vi "SFOAE-Create Swept Stimuli.vi"(0 "SFOAE Stim":T1, 5 "Data Folder":path, 9 "Fs (Hz)":dbl, 11 "error in (no error)":errorcluster) -> (4 "probe":dbl[](array[numeric]), 6 "suppressor":dbl[](array[numeric]), 8 "offset":i32, 10 "nfft":i32, 15 "error out":errorcluster)   [LabVIEW 2020]
uses:
  Typedefs/SFOAE-Stimulus Parameters.ctl
  Typedefs/SFOAE-Sweep Params.ctl
  epl-vi-lib/Utility VIs/Type Defs/Speaker ring.ctl
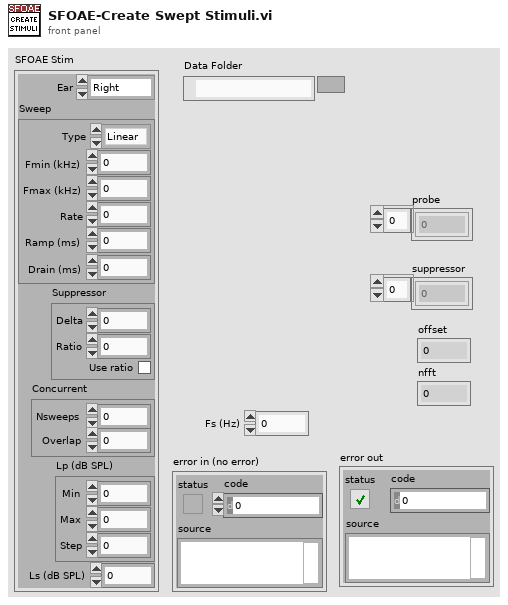
[diagram p1: front panel]
types:
  T1 = typedef "SFOAE-Stimulus Parameters.ctl" = cluster{"Ear":enum16{"Right", "Left"}, "Sweep":T2, "Suppressor":cluster{"Delta":dbl, "Ratio":dbl, "Use ratio":bool}, "Concurrent":cluster{"Nsweeps":i32, "Overlap":dbl}, "Ls (dB SPL)":dbl, "Lp (dB SPL)":cluster{"Min":dbl, "Max":dbl, "Step":dbl}}
  T2 = typedef "SFOAE-Sweep Params.ctl" = cluster{"Type":enum16{"Linear", "Log"}, "Fmin (kHz)":dbl, "Fmax (kHz)":dbl, "Rate":dbl, "Ramp (ms)":dbl, "Drain (ms)":dbl}
  T3 = typedef "Speaker ring.ctl" = enum16{"Right primary", "Right secondary", "Left primary", "Left secondary"}
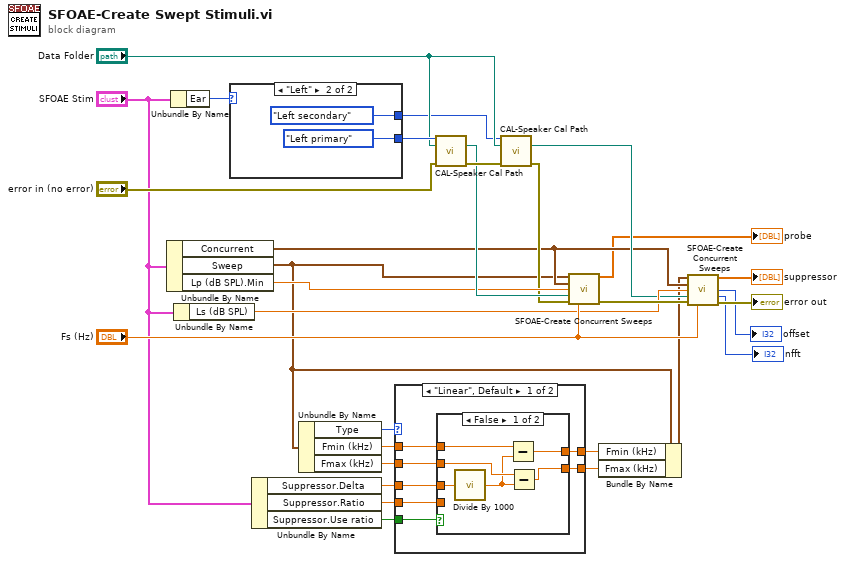
[diagram p0: block diagram]
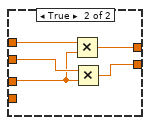
[diagram p2: hidden frame]
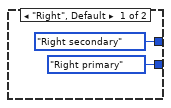
[diagram p4: hidden frame]
diagram:
  n1 = Unbundle By Name("SFOAE Stim") -> ("Concurrent"=w17:cluster{"Nsweeps":i32, "Overlap":dbl}, "Sweep"=w11:T2, "Lp (dB SPL).Min"=w23:dbl)
  n2 = Unbundle By Name("SFOAE Stim") -> ("Ear"=w30:enum16{"Right", "Left"})
  n3 = Unbundle By Name("SFOAE Stim") -> ("Ls (dB SPL)"=w19:dbl)
  n4 = case shown="\"Left\"" w30 {
    tunnel: [Speaker_ring."Right secondary" ("Speaker") Speaker_ring."Left secondary" ("Speaker")] -> w27
    tunnel: [Speaker_ring."Right primary" ("Speaker") Speaker_ring."Left primary" ("Speaker")] -> w29
    frame "Right", Default {
    }
    frame "Left" {
    }
  }
  n5 = Unbundle By Name("SFOAE Stim") -> ("Suppressor.Delta"=w7:dbl, "Suppressor.Ratio"=w4:dbl, "Suppressor.Use ratio"=w8:bool)
  n6 = Unbundle By Name(w11) -> ("Type"=w14:enum16{"Linear", "Log"}, "Fmin (kHz)"=w10:dbl, "Fmax (kHz)"=w9:dbl)
  n7 = case shown="\"Linear\", Default" w14 {
    tunnel: w10 -> [w41 _]
    tunnel: w9 -> [w39 _]
    tunnel: w8 -> [w40 _]
    tunnel: w7 -> [w38 _]
    tunnel: [w37 _] -> w6
    tunnel: [w36 _] -> w5
    tunnel: w4 -> [w35 _]
    frame "Linear", Default {
      n8 = case shown="False" w40 {
        tunnel: w41 -> [w47 w52]
        tunnel: w39 -> [w45 w50]
        tunnel: w38 -> [w44 w48]
        tunnel: [w46 w51] -> w37
        tunnel: [w43 w49] -> w36
        tunnel: w35 -> [_ _]
        frame False {
          n9 = call "Divide By 1000.vi"("X"=w44) -> ("X/1000"=w42:dbl)
          n10 = Subtract(x=w47, y=w42) -> (x-y=w46:dbl)
          n11 = Subtract(x=w45, y=w42) -> (x-y=w43:dbl)
        }
        frame True {
          n12 = Multiply(x=w52, y=w48) -> (x*y=w51:dbl)
          n13 = Multiply(x=w50, y=w48) -> (x*y=w49:dbl)
        }
      }
    }
    frame "Log" {
    }
  }
  n14 = call "CAL-Speaker Cal Path.vi"("Speaker"=w29, "Data Folder"="Data Folder", "error in (no error)"="error in (no error)") -> ("Cal Path"=w24:path, "error out"=w26:errorcluster)  [unwired: 11 in]
  n15 = call "CAL-Speaker Cal Path.vi"("Speaker"=w27, "Data Folder"="Data Folder", "error in (no error)"=w26) -> ("Cal Path"=w18:path, "error out"=w22:errorcluster)  [unwired: 11 in]
  n16 = call "SFOAE-Create Concurrent Sweeps.vi"("Sweep"=w11, "Concurrent"=w17, "Level (dB SPL)"=w23, "Cal File"=w24, "error in (no error)"=w22, "Fs (Hz)"="Fs (Hz)") -> ("sweep"=→"probe":dbl[], "error out"=w21:errorcluster)  [unwired: 6 in, 2 out]
  n17 = Bundle By Name(cluster=w11, "Fmin (kHz)"=w6, "Fmax (kHz)"=w5) -> (w13:T2)
  n18 = call "SFOAE-Create Concurrent Sweeps.vi"("Sweep"=w13, "Concurrent"=w17, "Level (dB SPL)"=w19, "Cal File"=w18, "error in (no error)"=w21, "Fs (Hz)"="Fs (Hz)") -> ("sweep"=→"suppressor":dbl[], "offset"=→"offset":i32, "nfft"=→"nfft":i32, "error out"=→"error out":errorcluster)  [unwired: 6 in]
